vi "Set Server Stop UE.vi"(10 "Server Stop":refnum<user-event>, 11 "OOP Server in":refnum<class "Temperature_server.lvclass">) -> (3 "OOP Server out":refnum<class "Temperature_server.lvclass">)   [LabVIEW 2019, in "Temperature_server.lvlib" / "Temperature_server.lvclass"]
uses:
  Temperature_server.lvclass
  Temperature_server.lvclass/Temperature_server.ctl
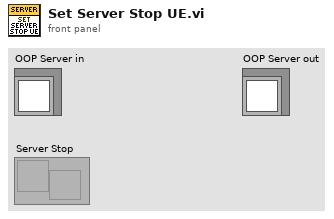
[diagram p1: front panel]
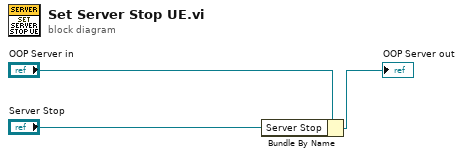
[diagram p0: block diagram]
diagram:
  n1 = Bundle By Name(cluster="OOP Server in", "Server Stop"="Server Stop") -> (→"OOP Server out":refnum<class "Temperature_server.lvclass">)
